vi "Dispose Buffer.vi"(8 "error in (no error)":errorcluster, 11 "Buffer":refnum<class "Buffer.lvclass">) -> (0 "error out":errorcluster, 3 "Buffer type":refnum<class "Buffer.lvclass">)   [LabVIEW 2017, in "DSF Core.lvlib" / "Buffer.lvclass"]
doc: "Disposes of the provided <b>Buffer</b>.\n\nThis will deallocate the pointer associated with the <b>Buffer</b>, so no further access of <b>Buffer</b> should be made."
uses:
  Buffer.lvclass
  C:/Git/DSF/LabVIEW-Memory/Source/Classes/Pointer/Pointer.lvclass
  LabVIEW-Memory/Source/Classes/Pointer/Pointer.lvclass
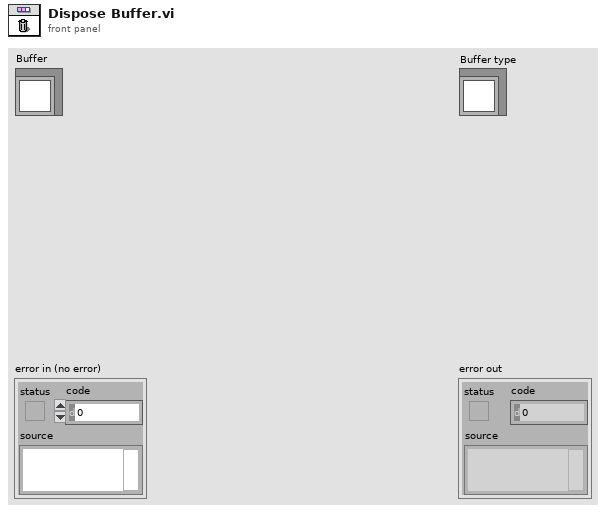
[diagram p1: front panel]
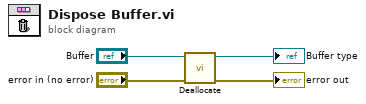
[diagram p0: block diagram]
diagram:
  n1 = call "Deallocate.vi"("error in (no error)"="error in (no error)", "Pointer in"="Buffer") -> ("error out"=→"error out":errorcluster, "Pointer out"=→"Buffer type":refnum<class "Buffer.lvclass">)  [unwired: 8 in]
